vi "SwitchChan.vi"(0 "reference in":refnum<class "Switch_Keysight_34934A.lvclass">, 1 "Matrix":T1=enum."M2L", 2 "Row":i32, 3 "Column":i32, 4 "State":bool, 5 "error in (no error)":errorcluster) -> (14 "reference in":refnum<class "Switch_Keysight_34934A.lvclass">, 19 "error out":errorcluster)   [LabVIEW 2022 SP3, in "Switch_Keysight_34934A.lvlib" / "Switch_Keysight_34934A.lvclass"]
uses:
  Switch_Keysight_34934A.lvclass
  Matrix.ctl
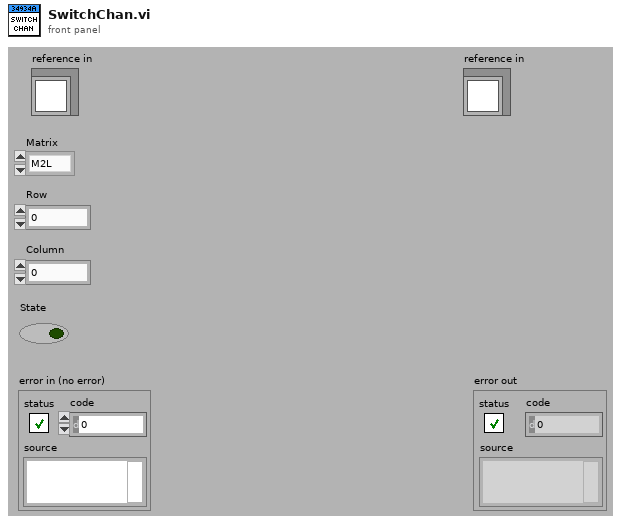
[diagram p1: front panel]
types:
  T1 = typedef "Switch_Keysight_34934A.lvlib/Switch_Keysight_34934A.lvclass/Matrix.ctl" = enum16{"M1H", "M2H", "M1L", "M2L"}
  T2 = typedef "Switch_Keysight_34934A.lvlib/Switch_Keysight_34934A.lvclass/ObjectAttributes.ctl" = cluster{"Config":T3, "VISA ref":refnum<visa-resource-name>, "M1H":bool[][], "M2H":bool[][], "M1L":bool[][], "M2L":bool[][], "route":string, "State":bool[], "StateModBit":bool[], "UpdateEvent":refnum<user-event>}
  T3 = typedef "Switch_Keysight_34934A.lvlib/Switch_Keysight_34934A.lvclass/Config.ctl" = cluster{"VISA":refnum<visa-resource-name>, "Slot":i32, "SwitchMap":cluster{"Name":string, "Route":string[], "UnRoute":string[], "Description":string, "Group":string, "IsGroup":bool}[], "Sim":bool}
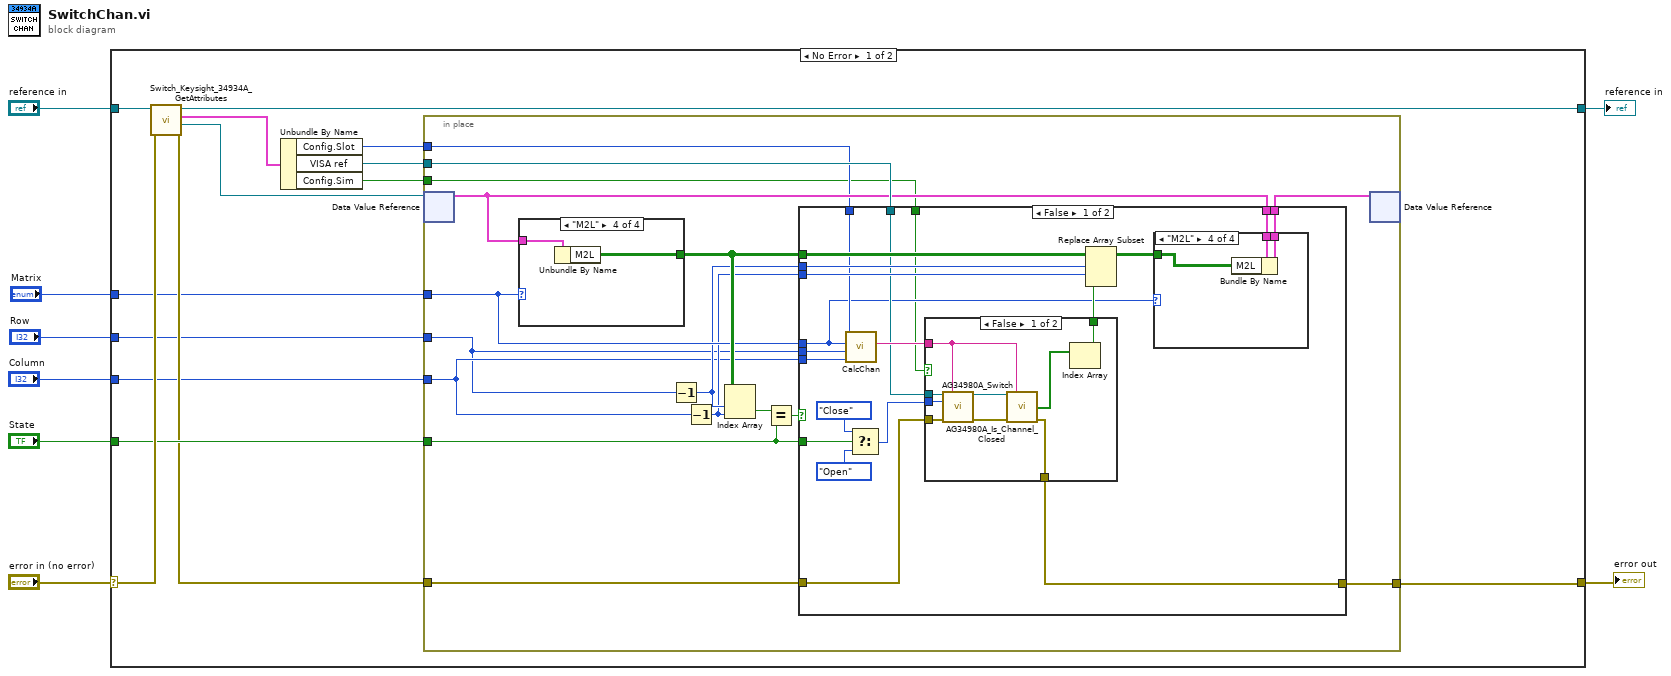
[diagram p0: block diagram]
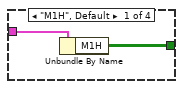
[diagram p2: hidden frame]
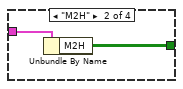
[diagram p3: hidden frame]
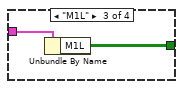
[diagram p4: hidden frame]
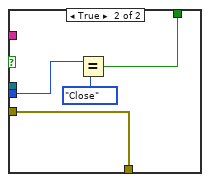
[diagram p5: hidden frame]
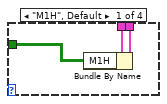
[diagram p6: hidden frame]
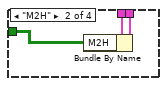
[diagram p7: hidden frame]
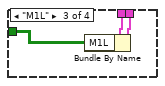
[diagram p8: hidden frame]
diagram:
  n1 = case shown="No Error" "error in (no error)" {
    selector: "error in (no error)" -> [w22 w95]
    tunnel: [w10 w95] -> w7
    tunnel: [w9 w94] -> w5
    tunnel: "reference in" -> [w20 w94]
    tunnel: "Row" -> [w14 _]
    tunnel: "Column" -> [w15 _]
    tunnel: "State" -> [w18 _]
    tunnel: "Matrix" -> [w13 _]
    frame No Error {
      n2 = call "Switch_Keysight_34934A_GetAttributes.vi"("error in (no error)"=w22, "reference in"=w20) -> ("error out"=w16:errorcluster, "DataRef"=w19:refnum<data-value>, "Data"=w21:T2, "reference out"=w9:refnum<class "Switch_Keysight_34934A.lvclass">)  [unwired: 6 in]
      n3 = Unbundle By Name(w21) -> ("Config.Slot"=w12:i32, "VISA ref"=w17:refnum<visa-resource-name>, "Config.Sim"=w11:bool)
      n4 = in-place {
        in-place-border: w18 -> [w35]
        in-place-border: w17 -> [w34]
        in-place-border: w16 -> [w33]
        in-place-border: [w32] -> w10
        in-place-border: w15 -> [w25]
        in-place-border: w14 -> [w24]
        in-place-border: w13 -> [w28]
        in-place-border: w12 -> [w29]
        in-place-border: w11 -> [w23]
        n5 = in-place-dvr #1(w19) -> (w31:T2)  [unwired: 1 out]
        n6 = case shown="\"M2L\"" w28 {
          tunnel: w31 -> [w40 w42 w44 w46]
          tunnel: [w39 w41 w43 w45] -> w30
          frame "M1H", Default {
            n7 = Unbundle By Name(w40) -> ("M1H"=w39:bool[][])
          }
          frame "M2H" {
            n8 = Unbundle By Name(w42) -> ("M2H"=w41:bool[][])
          }
          frame "M1L" {
            n9 = Unbundle By Name(w44) -> ("M1L"=w43:bool[][])
          }
          frame "M2L" {
            n10 = Unbundle By Name(w46) -> ("M2L"=w45:bool[][])
          }
        }
        n11 = Decrement(x=w24) -> (x-1=w27:i32)
        n12 = Decrement(x=w25) -> (x-1=w26:i32)
        n13 = Index Array(array=w30, index (row)=w27, index (col)=w26) -> (element=w37:bool)
        n14 = Equal?(x=w37, y=w35) -> (x = y?=w36:bool)
        n15 = case shown="False" w36 {
          tunnel: w31 -> [w66 w93]
          tunnel: [w65 w93] -> w38
          tunnel: w30 -> [w64 _]
          tunnel: w35 -> [w54 _]
          tunnel: w34 -> [w55 _]
          tunnel: w33 -> [w57 w92]
          tunnel: [w56 w92] -> w32
          tunnel: w27 -> [w63 _]
          tunnel: w26 -> [w62 _]
          tunnel: w29 -> [w61 _]
          tunnel: w28 -> [w49 _]
          tunnel: w24 -> [w60 _]
          tunnel: w25 -> [w59 _]
          tunnel: w23 -> [w47 _]
          frame False {
            n16 = call "CalcChan.vi"("Col"=w59, "Row"=w60, "Matrix"=w49, "Slot"=w61) -> ("Chan"=w58:string)  [unwired: 6 in, 1 out]
            n17 = Select(t=enum16{"Close", "Open"}."Close" ("Open/Close (0:Close)"), s=w54, f=enum16{"Close", "Open"}."Open" ("Open/Close (0:Close)")) -> (s? t:f=w51:enum16{"Close", "Open"})
            n18 = case shown="False" w47 {
              tunnel: w58 -> [w73 _]
              tunnel: w57 -> [w72 w79]
              tunnel: [w71 w79] -> w56
              tunnel: w55 -> [w70 _]
              tunnel: w51 -> [w69 w78]
              tunnel: [w67 w76] -> w50
              frame False {
                n19 = call "AG34980A_Switch.vi"("VISA resource name"=w70, "Channel List"=w73, "Open/Close (0:Close)"=w69, "error in (no error)"=w72) -> ("VISA resource name out"=w74:refnum<visa-resource-name>, "error out"=w75:errorcluster)  [unwired: 9 in, 1 out]
                n20 = call "AG34980A_Is_Channel_Closed.vi"("VISA resource name"=w74, "Channel List"=w73, "error in (no error)"=w75) -> ("Channel Status (Closed = True)"=w68:bool[], "error out"=w71:errorcluster)  [unwired: 10 in, 1 out]
                n21 = Index Array(array=w68) -> (element=w67:bool)  [unwired: 1 in]
              }
              frame True {
                n22 = Equal?(x=w78, y=enum16{"Close", "Open"}."Close" ("Open/Close (0:Close)")) -> (x = y?=w76:bool)
              }
            }
            n23 = Replace Array Subset(array=w64, new element=w50, index (row)=w63, index (col)=w62) -> (w48:bool[][])
            n24 = case shown="\"M2L\"" w49 {
              tunnel: w66 -> [w82 w85 w88 w91]
              tunnel: [w81 w84 w87 w90] -> w65
              tunnel: w48 -> [w80 w83 w86 w89]
              frame "M1H", Default {
                n25 = Bundle By Name(cluster=w82, "M1H"=w80) -> (w81:T2)
              }
              frame "M2H" {
                n26 = Bundle By Name(cluster=w85, "M2H"=w83) -> (w84:T2)
              }
              frame "M1L" {
                n27 = Bundle By Name(cluster=w88, "M1L"=w86) -> (w87:T2)
              }
              frame "M2L" {
                n28 = Bundle By Name(cluster=w91, "M2L"=w89) -> (w90:T2)
              }
            }
          }
          frame True {
          }
        }
        n29 = in-place-dvr #1(w38) -> ()  [unwired: 2 out]
      }
    }
    frame Error {
    }
  }
  "error out" <- w7
  "reference in" <- w5
